vi "MotionProfileSolver.vi"(8 "Max profiles":T3={"Max jerk"=100.0, "Max acceleration"=10.0, "Max Velocity"=10.0}, 9 "initalVelocity":dbl format="%#_13g", 10 "initalAccel":dbl format="%#_13g", 11 "Distance to go":dbl=10.0 format="%#_13g") -> (3 "TimeSegments":T1)   [LabVIEW 2014]
uses:
  Max profiles.ctl
  TimeSegments.ctl
  TimeSegment.ctl
panel:
  out "TimeAtEnd 2":dbl
  out "TimeAtEnd":dbl
  out "deltaX":dbl
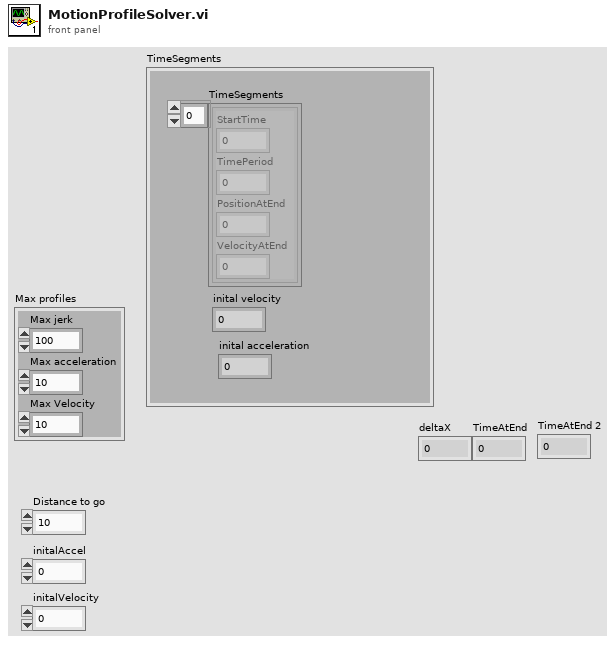
[diagram p1: front panel]
types:
  T1 = typedef "TimeSegments.ctl" = cluster{"TimeSegments":T2[], "inital velocity":dbl, "inital acceleration":dbl}
  T2 = typedef "TimeSegment.ctl" = cluster{"StartTime":dbl, "TimePeriod":dbl, "PositionAtEnd":dbl, "VelocityAtEnd":dbl}
  T3 = typedef "Max profiles.ctl" = cluster{"Max jerk":dbl, "Max acceleration":dbl, "Max Velocity":dbl}
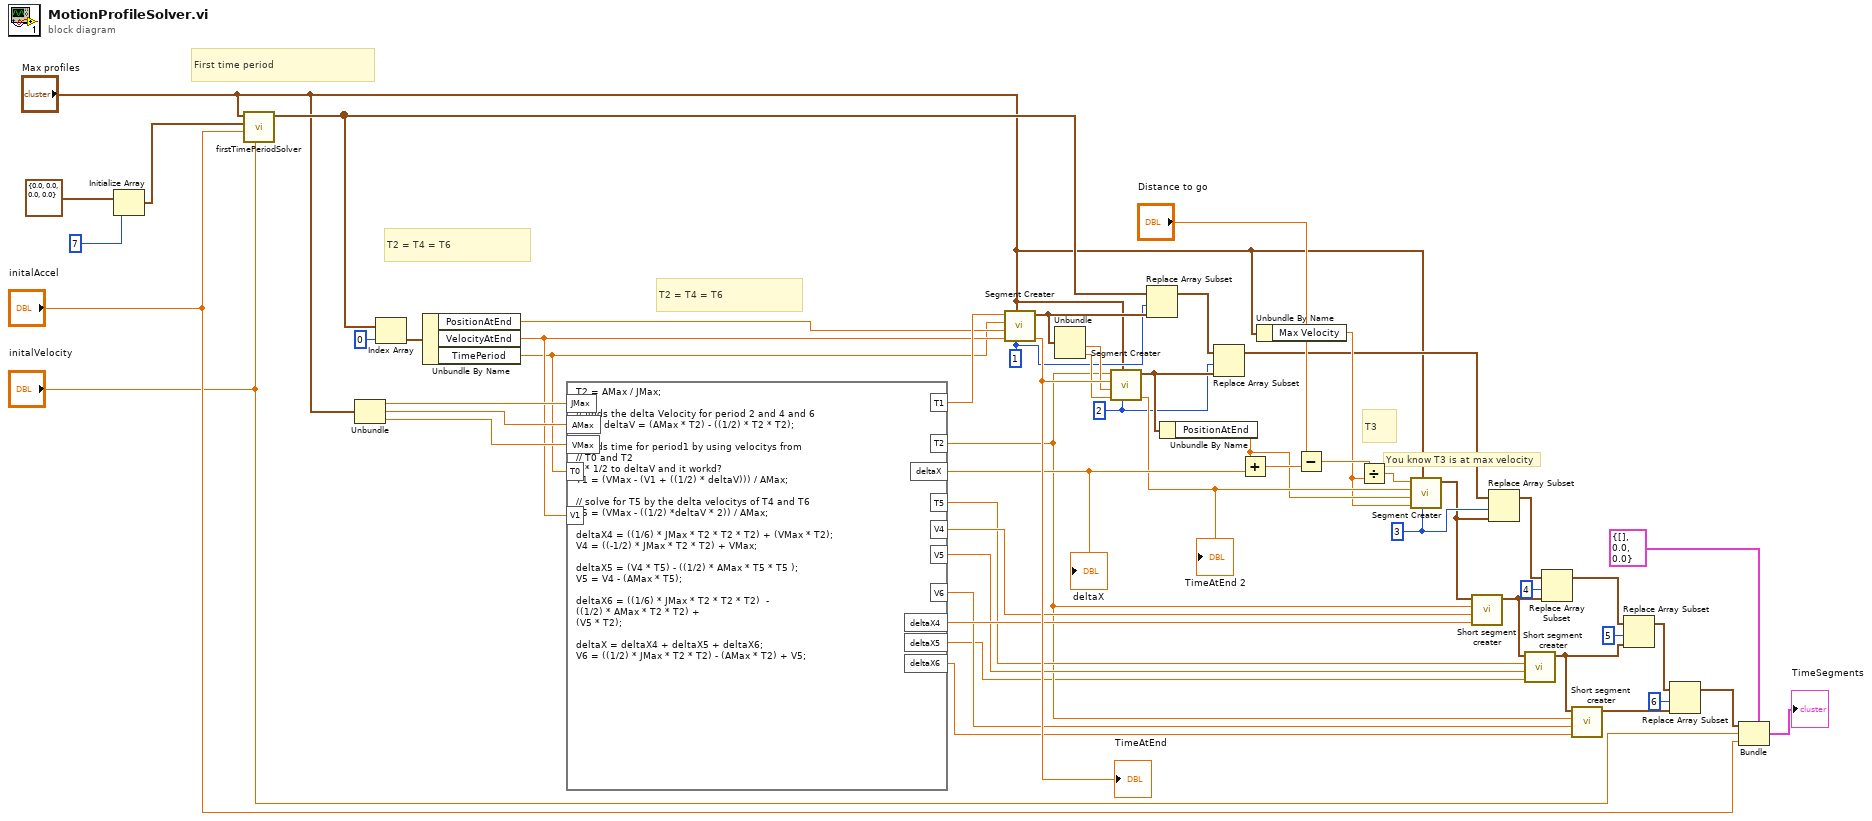
[diagram p0: block diagram]
diagram:
  w26 = i8 3 ("Time Period")
  w27 = i8 2 ("Time Period")
  w28 = i8 1 ("Time Period")
  # "You know T3 is at max velocity"
  # "T3"
  # "T2 = T4 = T6"
  # "T2 = T4 = T6"
  # "First time period"
  n1 = Initialize Array(T2 {"StartTime"=0.0, "TimePeriod"=0.0, "PositionAtEnd"=0.0, "VelocityAtEnd"=0.0} ("TimeSegment"), 7 ("dimension size")) -> (w54:T2[])
  n2 = call "firstTimePeriodSolver.vi"("initalVelocity"="initalVelocity", "initalAccel"="initalAccel", "Array in"=w54, "Max profiles"="Max profiles") -> ("Array out"=w44:T2[])  [unwired: 7 in]
  n3 = Unbundle("Max profiles") -> ("Max jerk"=w50:dbl, "Max acceleration"=w49:dbl, "Max Velocity"=w48:dbl)
  n4 = Index Array(array=w44, index=0) -> (element=w51:T2)
  n5 = Unbundle By Name(w51) -> ("PositionAtEnd"=w45:dbl, "VelocityAtEnd"=w46:dbl, "TimePeriod"=w38:dbl)
  n6 = formula code="T2 = AMax / JMax;\n\n// finds the delta Velocity for period 2 and 4 and 6\n float deltaV = (AMax * T2) - ((1/2) * T2 * T2);\n\n// finds time for period1 by using velocitys from\n// T0 and T2\n// * 1/2 to deltaV and it workd?\nT1 = (VMax - (V1 + ((1/2) * deltaV))) / AMax;\n\n// solve for T5 by the delta velocitys of T4 and T6\nT5 = (VMax - ((1/2) *deltaV * 2)) / AMax;\n\ndeltaX4 = ((1/6) * JMax * T2 * T2 * T2) + (VMax * T2);\nV4 = ((-1/2) * JMax * T2 * T2) + VMax;\n\ndeltaX5 = (V4 * T5) - ((1/2) * AMax * T5 * T5 );\nV5 = V4 - (AMax * T5);\n\ndeltaX6 = ((1/6) * JMax * T2 * T2 * T2)  -\n((1/2) * AMax * T2 * T2) +\n(V5 * T2);\n\ndeltaX = deltaX4 + deltaX5 + deltaX6;\nV6 = ((1/2) * JMax * T2 * T2) - (AMax * T2) + V5;"("JMax"=w50, "VMax"=w48, "T0"=w38, "V1"=w46, "AMax"=w49) -> ("T2"=w16:dbl, "T1"=w47:dbl, "T5"=w19:dbl, "V4"=w22:dbl, "V5"=w18:dbl, "deltaX"=w36:dbl, "deltaX4"=w21:dbl, "deltaX5"=w14:dbl, "deltaX6"=w13:dbl, "V6"=w15:dbl)
  "deltaX" <- w36
  n7 = call "Segment Creater.vi"("Time Segment"=w28, "Max profiles"="Max profiles", "Inital Segment Velocity"=w46, "Initial Segment Position"=w45, "StartTime"=w38, "TimePeriod"=w47) -> ("TimeAtEnd"=w42:dbl, "TimeSegment"=w43:T2)  [unwired: 4 in]
  "TimeAtEnd" <- w42
  n8 = Unbundle(w43) -> ("PositionAtEnd"=w41:dbl, "VelocityAtEnd"=w40:dbl)  [unwired: 2 out]
  n9 = call "Segment Creater.vi"("Time Segment"=w27, "Max profiles"="Max profiles", "Inital Segment Velocity"=w40, "Initial Segment Position"=w41, "StartTime"=w42, "TimePeriod"=w16) -> ("TimeAtEnd"=w31:dbl, "TimeSegment"=w37:T2)  [unwired: 4 in]
  "TimeAtEnd 2" <- w31
  n10 = Replace Array Subset(array=w44, new element=w43, index=w28) -> (w39:T2[])
  n11 = Unbundle By Name(w37) -> ("PositionAtEnd"=w30:dbl)
  n12 = Replace Array Subset(array=w39, new element=w37, index=w27) -> (w25:T2[])
  n13 = Add(x=w30, y=w36) -> (x+y=w35:dbl)
  n14 = Unbundle By Name("Max profiles") -> ("Max Velocity"=w29:dbl)
  n15 = Subtract(x="Distance to go", y=w35) -> (x-y=w33:dbl)
  n16 = Divide(x=w33, y=w29) -> (x/y=w32:dbl)
  n17 = call "Segment Creater.vi"("Time Segment"=w26, "Max profiles"="Max profiles", "Inital Segment Velocity"=w29, "Initial Segment Position"=w30, "StartTime"=w31, "TimePeriod"=w32) -> ("TimeSegment"=w23:T2)  [unwired: 4 in, 1 out]
  n18 = call "Short segment creater.vi"("deltaX"=w21, "Velocity"=w22, "Time Period"=w16, "LastTimeSegment"=w23) -> ("TimeSegment out"=w20:T2)  [unwired: 7 in]
  n19 = Replace Array Subset(array=w25, new element=w23, index=w26) -> (w17:T2[])
  n20 = call "Short segment creater.vi"("deltaX"=w14, "Velocity"=w18, "Time Period"=w19, "LastTimeSegment"=w20) -> ("TimeSegment out"=w11:T2)  [unwired: 7 in]
  n21 = Replace Array Subset(array=w17, new element=w20, index=4) -> (w12:T2[])
  n22 = call "Short segment creater.vi"("deltaX"=w13, "Velocity"=w15, "Time Period"=w16, "LastTimeSegment"=w11) -> ("TimeSegment out"=w9:T2)  [unwired: 7 in]
  n23 = Replace Array Subset(array=w12, new element=w11, index=5) -> (w10:T2[])
  n24 = Replace Array Subset(array=w10, new element=w9, index=6) -> (w3:T2[])
  n25 = Bundle(cluster=T1 {"TimeSegments"=[], "inital velocity"=0.0, "inital acceleration"=0.0} ("TimeSegments 2"), "TimeSegments"=w3, "inital velocity"="initalVelocity", "inital acceleration"="initalAccel") -> (→"TimeSegments":T1)
